vi "Start Acquisition.vi"(8 "error in (no error)":errorcluster, 11 "CCD in":refnum<class "CCD.lvclass">) -> (0 "error out":errorcluster, 3 "CCD out":refnum<class "CCD.lvclass">)   [LabVIEW 2018, in "CCD.lvclass"]
uses:
  CCD.lvclass
  CCD.lvclass/CCD.ctl
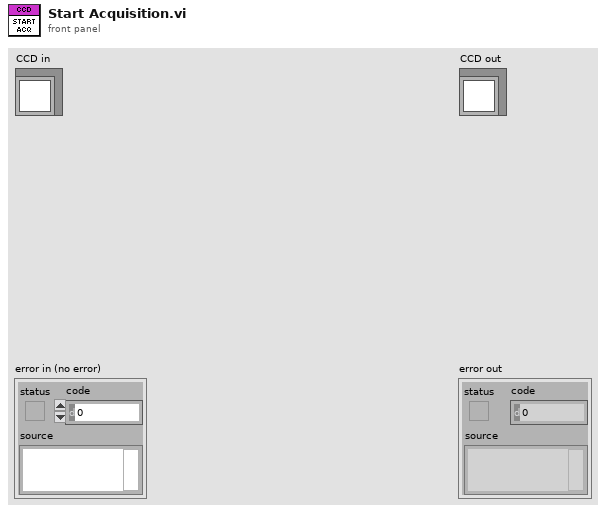
[diagram p1: front panel]
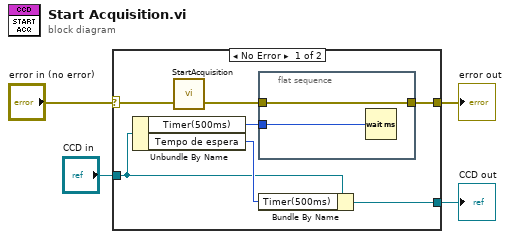
[diagram p0: block diagram]
diagram:
  n1 = case shown="No Error" "error in (no error)" {
    selector: "error in (no error)" -> [w11 w15]
    tunnel: [w6 w15] -> w2
    tunnel: [w8 w14] -> w1
    tunnel: "CCD in" -> [w9 w14]
    frame No Error {
      n2 = Unbundle By Name(w9) -> ("Timer(500ms)"=w5:u16, "Tempo de espera"=w10:u16)
      n3 = call <userlib>:"StartAcquisition.vi"("error in (no error)"=w11) -> ("error out"=w7:errorcluster)  [unwired: 1 in, 1 out]
      n4 = flat-sequence {
        tunnel: w7 -> [w13]
        tunnel: [w13] -> w6
        tunnel: w5 -> [w12]
        frame #0 {
          n5 = Wait (ms)(milliseconds to wait=w12) -> ()  [unwired: 1 out]
        }
      }
      n6 = Bundle By Name(cluster=w9, "Timer(500ms)"=w10) -> (w8:refnum<class "CCD.lvclass">)
    }
    frame Error {
    }
  }
  "error out" <- w2
  "CCD out" <- w1
